vi "Main.vi"() -> ()   [LabVIEW 2014]
uses:
  <vilib>/Stratom, Inc/X-Modules for myRIO/Type Defs/MXPChannel.ctl
  <vilib>/Stratom, Inc/X-CAN for myRIO (API)/X-CAN Class/Type Definitions/CAN_Speed.ctl
  <vilib>/Stratom, Inc/X-CAN for myRIO (API)/X-CAN Class/X-CAN.lvclass
panel:
  in  "Emission 3":bool
  in  "Periode chgt Img":u8[](array[numeric])=[10, 20, 0, 0, 0, 0, 15, 0]
  in  "Periode chgt image (en n x 20 ms) :":u8[](array[numeric])=[5, 5, 10, 10, 2, 8, 15, 15]
  in  "Num Img Proc":u8[](array[numeric])=[4, 14, 0, 0, 0, 0, 28, 0]
  in  "Numéro Image Process (-1 !!!!) :":u8[](array[numeric])=[8, 16, 12, 18, 20, 2, 22, 10]
  in  "Emission 2":bool
  in  "Crédit :":u8=5
  in  "Numéro Process [1..16] :":u8=15 max=16 step=1
  in  "Exploitation :":bool
  in  "Ack Piece :":bool
  in  "Emission":bool
  in  "Periode affichage 2 images [0 .. 255] x 35ms :":u8=20
  in  "Periode clignottement  [0 .. 255] x 35ms :":u8
  in  "Vitesse volet [1 .. 255] ms :":u8=1 min=1 step=1
  in  "Type volet :":u16(ring) items=["Aucun", "Ouvrant gauche", "Ouvrant droite", "Ouvrant central", "Fermant gauche", "Fermant droite", "Fermant central"]
  in  "Page Haute :":bool=TRUE
  in  "Num Image [1..32] :":u8=30 min=1 max=32 step=1
  in  "Val luminosité [0..255] :":u8
  in  "Commande à executer :":u16(ring)=1 items=["Mise à jour Luminosité", "Appel Image", "Appel Image + Volet", "Affichage Page Basse (non imp)", "Affichage Page Haute (non imp)", "Mise à jour clignottement", "Affichage 2 images (Periode)"]
  in  "Num Image [1 ... 32]":u8=16 min=1 max=32 step=1
  in  "Lec":bool
  out "Data":u8 format="%x"
  in  "Adr":u16=112 format="%x"
  out "Etat Emi EEp :":u16(slide)=512 scale=0.0..512.0
  in  "Emi Image EEp":bool
  out "Etat Lecture :":string="Lecture OK"
  in  "Lec Fic BMP":bool
  in  "Chemin d'acces fichiers sur clé MyRIO":path=path "u:/J1942_16c_2.bmp"
  in  "Stop Button":bool
  # "Appel Commandes asynchrones :"
  # "Status Paiement :"
  # "Transfert d'images (128x32pix 16 couleurs) vers la cible :"
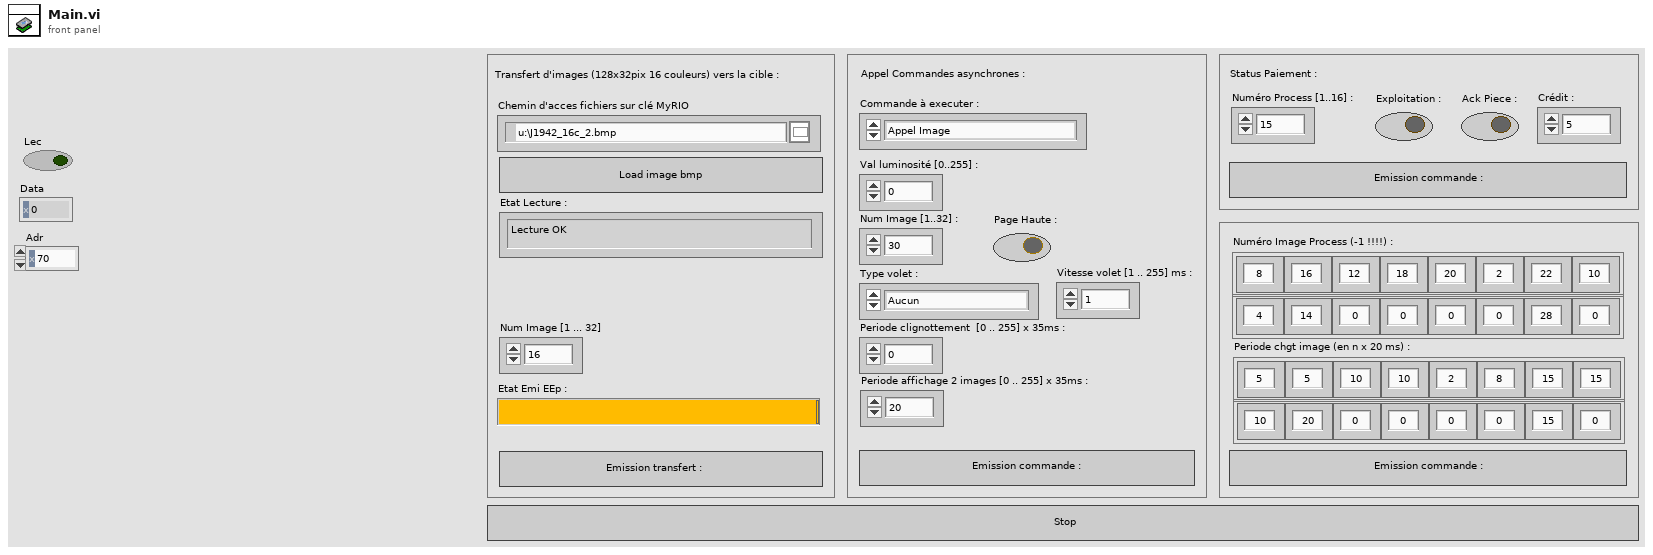
[diagram p1: front panel]
types:
  T1 = typedef "MXPChannel.ctl" = enum16{"A/MXP", "B/MXP"}
  T2 = typedef "X-CAN.lvclass/CAN_Speed.ctl" = u8
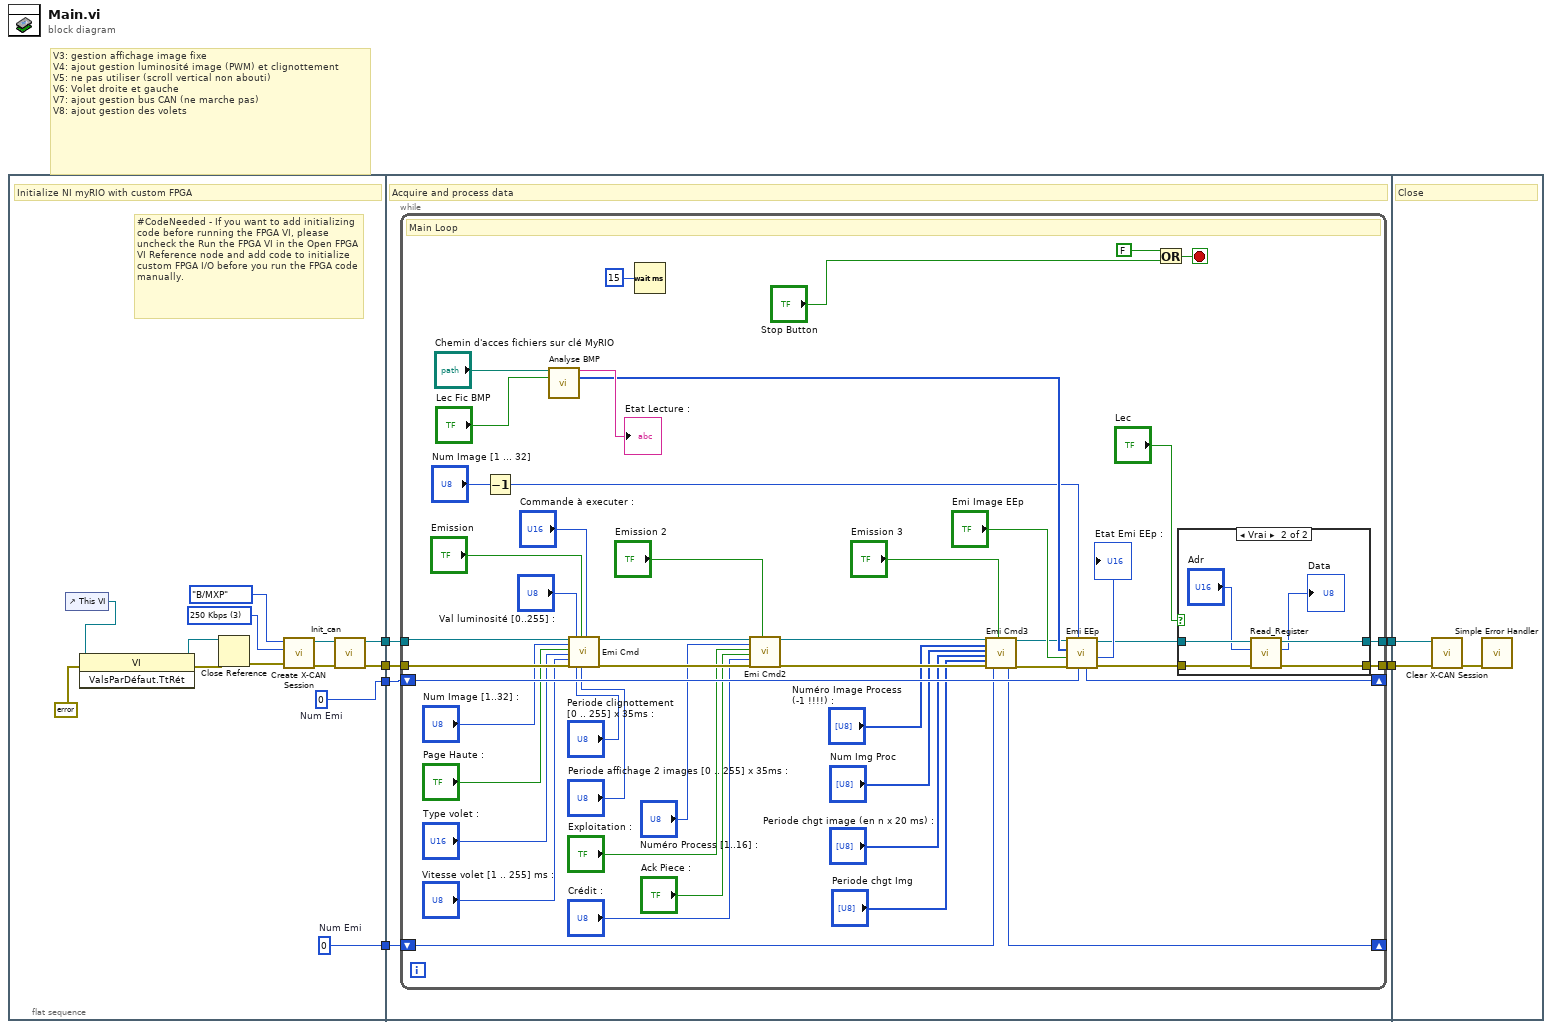
[diagram p0: block diagram]
diagram:
  # "V3: gestion affichage image fixe\nV4: ajout gestion luminosité image (PWM) et clignottement\nV5: ne pas utiliser (scroll vertical non abouti)\nV6: Volet droite et gauche\nV7: ajout gestion bus CAN (ne marche pas)\nV8: ajout gestion des volets"
  n1 = flat-sequence {
    tunnel: [w11] -> w6
    tunnel: [w10] -> w3
    tunnel: [w8] -> w2
    tunnel: [w7] -> w1
    tunnel: w6 -> [w25]
    tunnel: [w24] -> w5
    tunnel: [w23] -> w4
    tunnel: w3 -> [w22]
    tunnel: w2 -> [w21]
    tunnel: w1 -> [w20]
    tunnel: w5 -> [w83]
    tunnel: w4 -> [w82]
    frame #0 {
      w7 = u8 0  # Num Emi
      w10 = u16 0  # Num Emi
      w13 = T2 3 items=["125 Kbps"=7, "250 Kbps"=3, "500 Kbps"=1, "1000 Kbps"=0, "95.238 Kbps"=6] ("CAN Speed [Kbps]")
      # "#CodeNeeded - If you want to add initializing code before running the FPGA VI, please uncheck the Run the FPGA VI in the Open FPGA VI Reference node and add code to initialize custom FPGA I/O before you run the FPGA code manually."
      # "Initialize NI myRIO with custom FPGA"
      n2 = control-ref of="This VI"() -> (w9:refnum<vi>)
      n3 = invoke class="VI" method="ValsParDéfaut.TtRét"(reference=w9, error in=errorcluster {"status"=FALSE, "code"=0, "source"=""} ("error in (no error)")) -> (reference out=w16:refnum<vi>, error out=w15:errorcluster)  [unwired: 1 in, 1 out]
      n4 = Close Reference(reference=w16, error in (no error)=w15) -> (error out=w17:errorcluster)
      n5 = call <vilib>:"Create X-CAN Session.vi"("error in (no error)"=w17, "CAN Speed [Kbps]"=w13, "MXP Channel"=MXPChannel."B/MXP") -> ("error out"=w19:errorcluster, "X-CAN Session out"=w18:refnum<class "X-CAN.lvclass">)  [unwired: 7 in]
      n6 = call "Init_can.vi"("entrée d'erreur (pas d'erreur)"=w19, "X-CAN en entrée"=w18) -> ("sortie d'erreur"=w8:errorcluster, "X-CAN en sortie"=w11:refnum<class "X-CAN.lvclass">)  [unwired: 8 in]
    }
    frame #1 {
      # "Acquire and process data"
      n7 = while {
        tunnel: w25 -> [w54]
        tunnel: [w59] -> w24
        tunnel: [w58] -> w23
        shift-right: [w63] -> _
        shift-left: w22 -> [w64]
        tunnel: w21 -> [w53]
        shift-right: [w31] -> _
        shift-left: w20 -> [w32]
        stop <- w72 stop-if-true
        # "Main Loop"
        n8 = Decrement(x="Num Image [1 ... 32]") -> (x-1=w55:u8)
        n9 = call "Analyse BMP.vi"("Chemin d'acces"="Chemin d'acces fichiers sur clé MyRIO", "Lec Fic Midi"="Lec Fic BMP") -> ("Chaîne"=→"Etat Lecture :":string, "Matrix"=w67:u8[])  [unwired: 12 in]
        n10 = call "Emi Cmd.vi"("X-CAN en entrée"=w54, "Num Image [1..32] :"="Num Image [1..32] :", "Page Haute :"="Page Haute :", "Type volet :"="Type volet :", "Vitesse volet [1 .. 255] ms :"="Vitesse volet [1 .. 255] ms :", "entrée d'erreur (pas d'erreur)"=w53, "Val luminosité :"="Val luminosité [0..255] :", "Periode clignottement"="Periode clignottement  [0 .. 255] x 35ms :", "Emission"="Emission", "Periode affichage 2 images"="Periode affichage 2 images [0 .. 255] x 35ms :", "Commande à executer :"="Commande à executer :") -> ("X-CAN en sortie"=w43:refnum<class "X-CAN.lvclass">, "sortie d'erreur"=w42:errorcluster)  [unwired: 7 in]
        n11 = Wait (ms)(milliseconds to wait=u32 15) -> ()  [unwired: 1 out]
        n12 = call "Emi Cmd2.vi"("X-CAN en entrée"=w43, "Numéro Process [0..16] :"="Numéro Process [1..16] :", "Exploitation :"="Exploitation :", "Ack Piece :"="Ack Piece :", "Crédit :"="Crédit :", "entrée d'erreur (pas d'erreur)"=w42, "Emission"="Emission 2") -> ("X-CAN en sortie"=w36:refnum<class "X-CAN.lvclass">, "sortie d'erreur"=w34:errorcluster)  [unwired: 11 in]
        n13 = call "Emi Cmd3.vi"("X-CAN en entrée"=w36, "Numéro Image Attente"="Numéro Image Process (-1 !!!!) :", "Num Img Proc"="Num Img Proc", "Durée Img Proc"="Periode chgt image (en n x 20 ms) :", "Durée process"="Periode chgt Img", "entrée d'erreur (pas d'erreur)"=w34, "Num Emi In"=w32, "Emission"="Emission 3") -> ("Num Emi  Out"=w31:u8, "X-CAN en sortie"=w35:refnum<class "X-CAN.lvclass">, "sortie d'erreur"=w33:errorcluster)  [unwired: 9 in]
        n14 = call "Emi EEp.vi"("Num Emi In"=w64, "Num Image"=w55, "entrée d'erreur"=w33, "Emi Image EEp"="Emi Image EEp", "Matrix en entrée"=w67, "X-CAN en entrée"=w35) -> ("sortie d'erreur"=w60:errorcluster, "Etat Emi EEp"=→"Etat Emi EEp :":u16, "X-CAN en sortie"=w61:refnum<class "X-CAN.lvclass">, "Num Emi Out"=w63:u16)  [unwired: 2 in]
        n15 = Or(x=FALSE, y="Stop Button") -> (x .or. y?=w72:bool)
        n16 = case shown="Vrai" "Lec" {
          tunnel: w61 -> [w75 w81]
          tunnel: w60 -> [w74 w80]
          tunnel: [w75 w79] -> w59
          tunnel: [w74 w78] -> w58
          frame False {
          }
          frame True {
            n17 = call <vilib>:"Read_Register.vi"("error in"=w80, "Register"="Adr", "X-CAN Session in"=w81) -> ("error out"=w78:errorcluster, "Read Byte"=→"Data":u8, "X-CAN Session out"=w79:refnum<class "X-CAN.lvclass">)  [unwired: 6 in]
          }
        }
      }
    }
    frame #2 {
      # "Close"
      n18 = call <vilib>:"Clear X-CAN Session.vi"("error in (no error)"=w82, "X-CAN Session in"=w83) -> ("error out"=w84:errorcluster)  [unwired: 9 in]
      n19 = call <vilib>:"Simple Error Handler.vi"("error in (no error)"=w84) -> ()  [unwired: 4 in, 5 out]
    }
  }
